vi "setTensao.vi"(5 "Corrente":dbl, 7 "Ponto":i32, 8 "error in (no error)":errorcluster, 9 "Pontos":dbl, 10 "Tensão máxima":dbl, 11 "delay(ms)":dbl) -> (0 "error out":errorcluster, 2 "output voltage":dbl)   [LabVIEW 2012]
uses:
  <instrlib>/Agilent 6XXX Series/Agilent 6XXX Series.lvlib
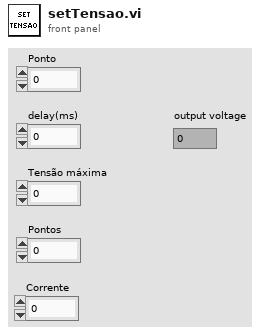
[diagram p1: front panel]
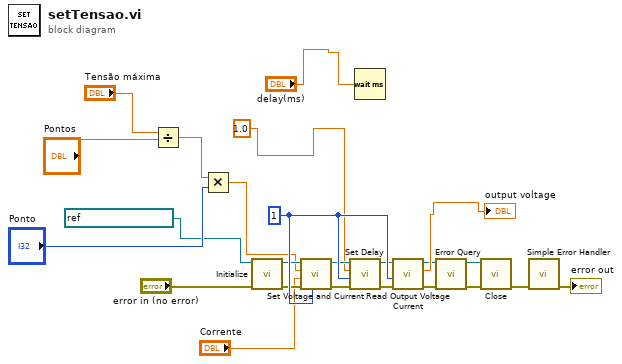
[diagram p0: block diagram]
diagram:
  w20 = u8 1 ("channel (1)")
  n1 = Divide(x="Tensão máxima", y="Pontos") -> (x/y=w19:dbl)
  n2 = Multiply(x=w19, y="Ponto") -> (x*y=w7:dbl)
  n3 = call <instrlib>:"Initialize.vi"("error in (no error)"="error in (no error)", "VISA resource name"=refnum<visa-resource-name> "GPIB0::5::INSTR") -> ("error out"=w13:errorcluster, "VISA resource name out"=w14:refnum<visa-resource-name>)  [unwired: 8 in]
  n4 = call <instrlib>:"Set Voltage and Current.vi"("channel (1)"=w20, "error in (no error)"=w13, "current (0 A)"="Corrente", "voltage (0 V)"=w7, "VISA resource name"=w14) -> ("error out"=w9:errorcluster, "VISA resource name out"=w8:refnum<visa-resource-name>)  [unwired: 5 in]
  n5 = call <instrlib>:"Set Delay.vi"("error in (no error)"=w9, "channel (1)"=w20, "delay (0 s)"=1.0, "VISA resource name"=w8) -> ("error out"=w5:errorcluster, "VISA resource name out"=w6:refnum<visa-resource-name>)  [unwired: 6 in]
  n6 = Wait (ms)(milliseconds to wait="delay(ms)") -> ()  [unwired: 1 out]
  n7 = call <instrlib>:"Read Output Voltage Current.vi"("error in (no error)"=w5, "channel (1)"=w20, "VISA resource name"=w6) -> ("error out"=w11:errorcluster, "output voltage"=→"output voltage":dbl, "VISA resource name out"=w10:refnum<visa-resource-name>)  [unwired: 5 in, 1 out]
  n8 = call <instrlib>:"Error Query.vi"("error in (no error)"=w11, "VISA resource name"=w10) -> ("error out"=w16:errorcluster, "VISA resource name out"=w15:refnum<visa-resource-name>)  [unwired: 6 in, 2 out]
  n9 = call <instrlib>:"Close.vi"("error in (no error)"=w16, "VISA resource name"=w15) -> ("error out"=w17:errorcluster)  [unwired: 9 in]
  n10 = call <vilib>:"Simple Error Handler.vi"("error in (no error)"=w17) -> ("error out"=→"error out":errorcluster)  [unwired: 4 in, 4 out]
